vi "Process Result.vi"(8 "error in (no error)":errorcluster, 9 "Acknowledge":bool, 10 "Result in":refnum<class "Acquired Result.lvclass">, 11 "Process Object in":refnum<class "Process Object.lvclass">) -> (0 "error out":errorcluster, 3 "Process Object out":refnum<class "Process Object.lvclass">)   [LabVIEW 2019, in "Process Object.lvclass"]
uses:
  Process Object.lvclass
  C:/GitHub/LabActor/Worker/Worker.lvclass
  C:/Program Files/National Instruments/LabVIEW 2019/vi.lib/ActorFramework/Actor/Actor.lvclass
  NHMFL_Core/Libraries/Instruments/Results/Acquired Result/Acquired Result.lvclass
  Worker/Worker.lvclass/Worker.ctl
  NHMFL_Core/Libraries/Instruments/Instrument Driver/Worker State.ctl
  <vilib>/ActorFramework/Actor/Actor.lvclass/Actor.ctl
  Controllers/Process Controller Messages/Update Plots Msg/Update Plots Msg.lvclass/Update Plots Msg.ctl
  <vilib>/ActorFramework/Message Enqueuer/Message Enqueuer.lvclass/Message Enqueuer.ctl
  Controllers/Process Controller Messages/Acknowledge Post Process Msg/Acknowledge Post Process Msg.lvclass/Acknowledge Post Process Msg.ctl
  Template Module/Write State.vi
  Template Module/Read State.vi
  <vilib>/ActorFramework/Message Enqueuer/Enqueue.vi
  Controllers/Process Controller Messages/Update Plots Msg/Update Plots Msg.lvclass
  C:/Program Files/National Instruments/LabVIEW 2019/vi.lib/ActorFramework/Message/Message.lvclass
  Controllers/Process Controller Messages/Acknowledge Post Process Msg/Acknowledge Post Process Msg.lvclass
  <vilib>/ActorFramework/Message Priority Queue/Priority Enqueue.vi
  <vilib>/ActorFramework/Actor/Actor.lvclass
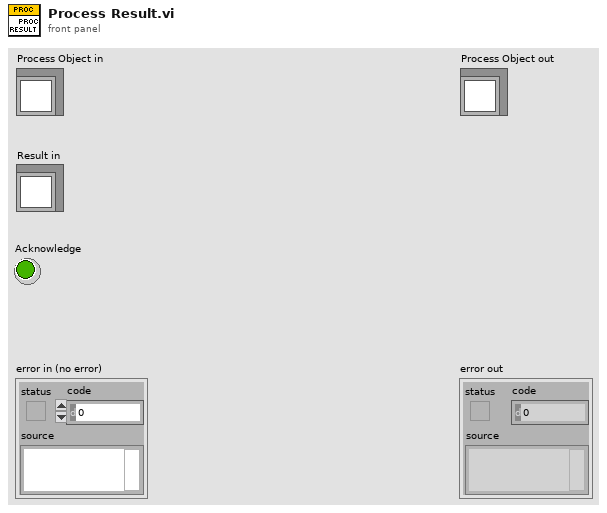
[diagram p1: front panel]
types:
  T1 = typedef "Worker State.ctl" = enum16{"Idle", "Starting", "Working", "Stopping"}
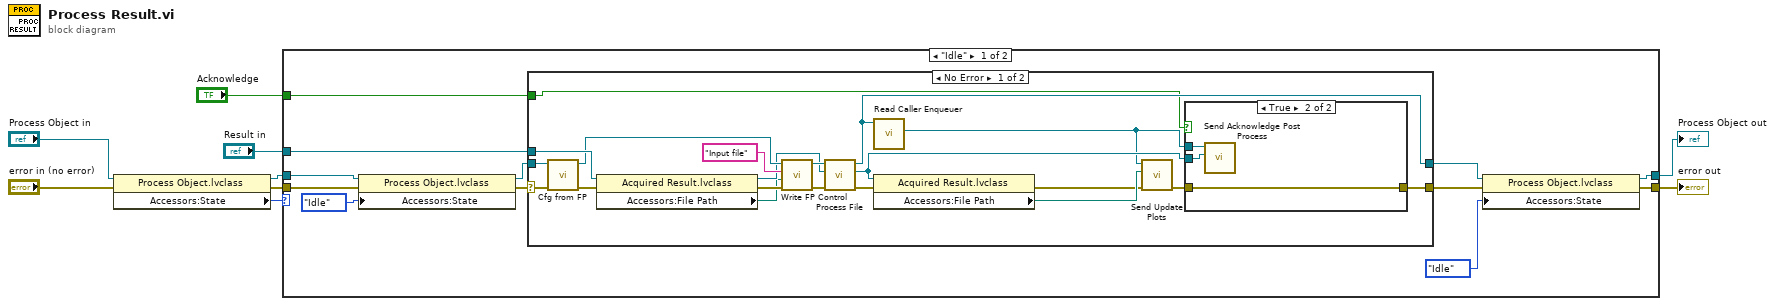
[diagram p0: block diagram]
diagram:
  n1 = property class="Process Object.lvclass"(reference="Process Object in", error in="error in (no error)") -> (reference out=w2:refnum<class "Process Object.lvclass">, error out=w4:errorcluster, "Accessors:State"=w1:T1)
  n2 = case shown="\"Idle\"" w1 {
    tunnel: [w13 w49] -> w8
    tunnel: [w11 w48] -> w7
    tunnel: "Result in" -> [w20 _]
    tunnel: "Acknowledge" -> [w19 _]
    tunnel: w4 -> [w18 w49]
    tunnel: w2 -> [w16 w48]
    frame "Idle" {
      n3 = property class="Process Object.lvclass"(reference=w16, error in=w18, "Accessors:State"=Worker_State."Idle" ("State")) -> (reference out=w15:refnum<class "Process Object.lvclass">, error out=w17:errorcluster)
      n4 = case shown="No Error" w17 {
        selector: w17 -> [w35 w47]
        tunnel: [w38 w47] -> w21
        tunnel: [w39 w46] -> w12
        tunnel: w15 -> [w37 w46]
        tunnel: w20 -> [w41 _]
        tunnel: w19 -> [w29 _]
        frame No Error {
          n5 = call-dynamic "Cfg from FP.vi"("error in (no error)"=w35, "Measure Object in"=w37) -> ("error out"=w36:errorcluster, "Measure Object out"=w34:refnum<class "Process Object.lvclass">)  [unwired: 8 in]
          n6 = property class="Acquired Result.lvclass"(reference=w41, error in=w36) -> (reference out=w28:refnum<class "Acquired Result.lvclass">, error out=w31:errorcluster, "Accessors:File Path"=w27:path)
          n7 = call-dynamic "Write FP Control.vi"("error in (no error)"=w31, "Control Value"=w27, "Control Name"="Input file", "Measure Object in"=w34) -> ("error out"=w30:errorcluster, "Measure Object out"=w33:refnum<class "Process Object.lvclass">)  [unwired: 6 in]
          n8 = call-dynamic "Process File.vi"("error in (no error)"=w30, "Result in"=w28, "Process Object in"=w33) -> ("error out"=w23:errorcluster, "Result out"=w40:refnum<class "Acquired Result.lvclass">, "Process Object out"=w39:refnum<class "Process Object.lvclass">)  [unwired: 6 in]
          n9 = call <vilib>:"Read Caller Enqueuer.vi"("Actor"=w39) -> ("Caller Enqueuer"=w24:refnum<class "Message Enqueuer.lvclass">)  [unwired: 10 in]
          n10 = property class="Acquired Result.lvclass"(reference=w40, error in=w23) -> (error out=w25:errorcluster, "Accessors:File Path"=w26:path)  [unwired: 1 out]
          n11 = call "Send Update Plots.vi"("error in (no error)"=w25, "File Path"=w26, "Message Enqueuer"=w24) -> ("error out"=w22:errorcluster)  [unwired: 7 in, 1 out]
          n12 = case shown="True" w29 {
            tunnel: w40 -> [_ w45]
            tunnel: w22 -> [w42 w43]
            tunnel: [w42 w43] -> w38
            tunnel: w24 -> [_ w44]
            frame False {
            }
            frame True {
              n13 = call "Send Acknowledge Post Process.vi"("Ack Result"=w45, "Message Enqueuer"=w44) -> ()  [unwired: 8 in, 2 out]
            }
          }
        }
        frame Error {
        }
      }
      n14 = property class="Process Object.lvclass"(reference=w12, error in=w21, "Accessors:State"=Worker_State."Idle" ("State")) -> (reference out=w11:refnum<class "Process Object.lvclass">, error out=w13:errorcluster)
    }
    frame "Working", Default {
    }
  }
  "error out" <- w8
  "Process Object out" <- w7
